vi "Untitled 1.vi"() -> ()   [LabVIEW 2015]
panel:
  in  "Signal Input":bool
  out "max(x,y)":dbl
  out "Stable":bool
  out "Out":dbl
  in  "Slide":dbl(slide) scale=-800.0..800.0
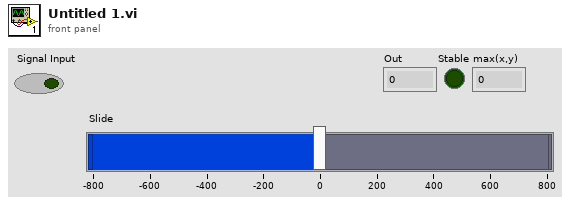
[diagram p1: front panel]
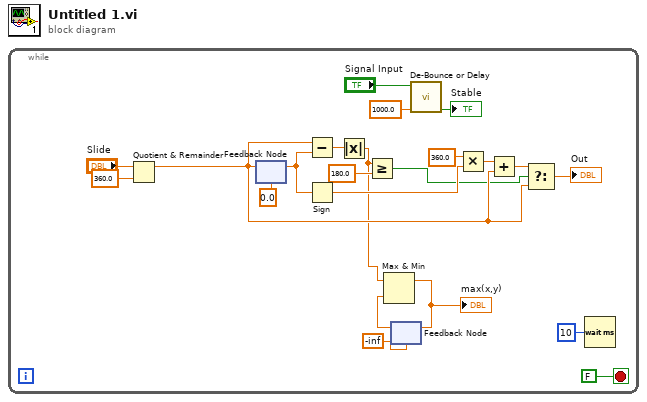
[diagram p0: block diagram]
diagram:
  n1 = while {
    stop <- FALSE stop-if-true
    n2 = Quotient & Remainder(x="Slide", y=360.0) -> (x-y*floor(x/y)=w9:dbl)  [unwired: 1 out]
    n3 = feedback #1(0.0) -> (w19:dbl)
    n4 = feedback-in #1(w9) -> ()
    n5 = Subtract(x=w9, y=w19) -> (x-y=w21:dbl)
    n6 = Sign(1:w19) -> (0:w15:dbl)
    n7 = Absolute Value(x=w21) -> (abs(x)=w6:dbl)
    n8 = Greater Or Equal?(x=w6, y=180.0) -> (x >= y?=w2:bool)
    n9 = feedback #2(-inf) -> (w4:dbl)
    n10 = Max & Min(x=w6, y=w4) -> (max(x,y)=w5:dbl)  [unwired: 1 out]
    "max(x,y)" <- w5
    n11 = feedback-in #2(w5) -> ()
    n12 = call <userlib>:"De-Bounce or Delay.vi"("Eval Period (sec)"=1000.0, "Signal Input"="Signal Input") -> ("Stable"=→"Stable":bool)  [unwired: 9 in]
    n13 = Multiply(x=360.0 ("y"), y=w15) -> (x*y=w17:dbl)
    n14 = Add(x=w17, y=w9) -> (x+y=w18:dbl)
    n15 = Select(t=w18, s=w2, f=w9) -> (s? t:f=→"Out":dbl)
    n16 = Wait (ms)(milliseconds to wait=u32 10) -> ()  [unwired: 1 out]
  }
